vi "AuthSrpInitiationRequest_Parse.vi"(8 "error in (no error)":errorcluster, 11 "Message":T5) -> (0 "error out":errorcluster, 1 "Body":T1, 2 "Header":T3, 3 "AuthSrpInitiationRequest":T2)   [LabVIEW 2017]
uses:
  <vilib>/addons/InsightCM/MessageBus/Base/controls/Message.ctl
  <vilib>/addons/InsightCM/MessageBus/Base/controls/MessageHeader.ctl
  <vilib>/addons/InsightCM/MessageBus/Base/controls/KeyValuePair.ctl
  <vilib>/addons/InsightCM/MessageBus/MessageLibrary/Authentication/controls/AuthSrpInitiationRequest.ctl
  <vilib>/addons/InsightCM/MessageBus/MessageLibrary/Authentication/controls/AuthSrpInitiationRequestBody.ctl
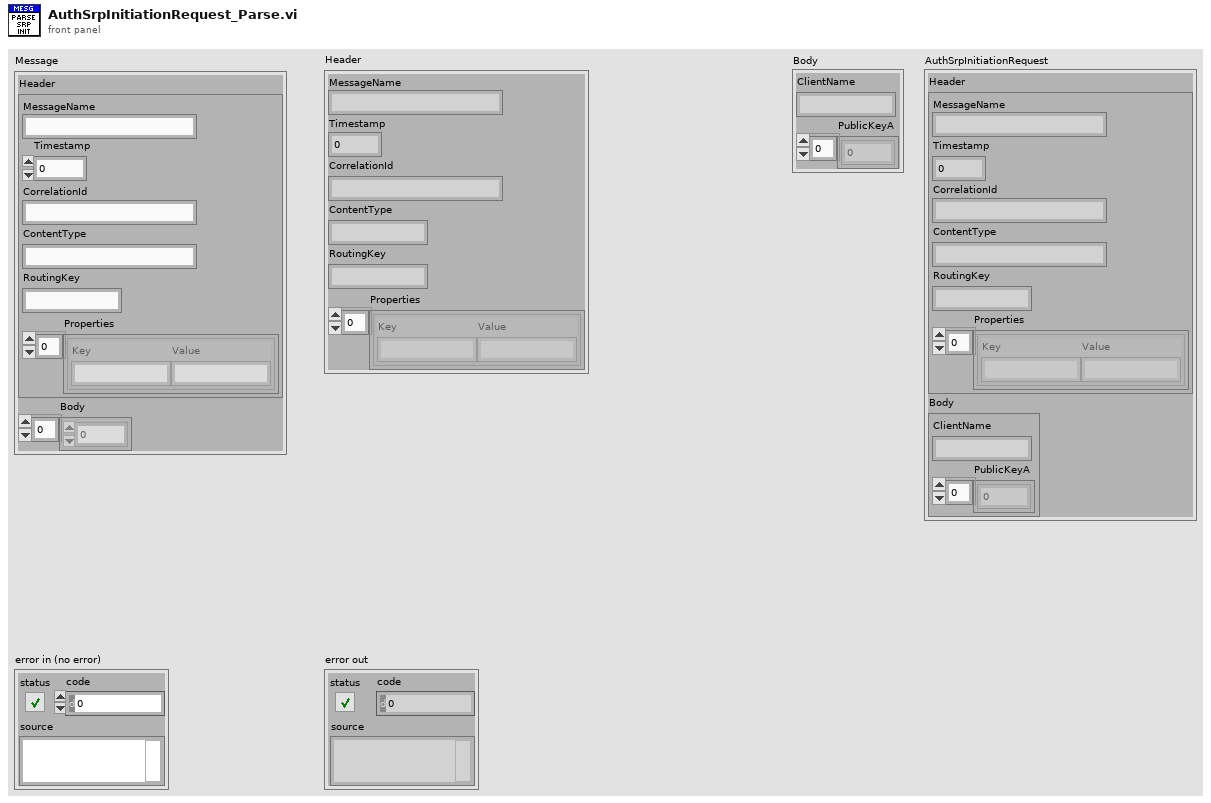
[diagram p1: front panel]
types:
  T1 = typedef "AuthSrpInitiationRequestBody.ctl" = cluster{"ClientName":string, "PublicKeyA":u8[]}
  T2 = typedef "AuthSrpInitiationRequest.ctl" = cluster{"Header":T3, "Body":T1}
  T3 = typedef "MessageHeader.ctl" = cluster{"MessageName":string, "Timestamp":i64, "CorrelationId":string, "ContentType":string, "RoutingKey":string, "Properties":T4[]}
  T4 = typedef "KeyValuePair.ctl" = cluster{"Key":string, "Value":string}
  T5 = typedef "Message.ctl" = cluster{"Header":T3, "Body":u8[]}
  T6 = cluster{"ClientName":string, "PublicKeyA":string}
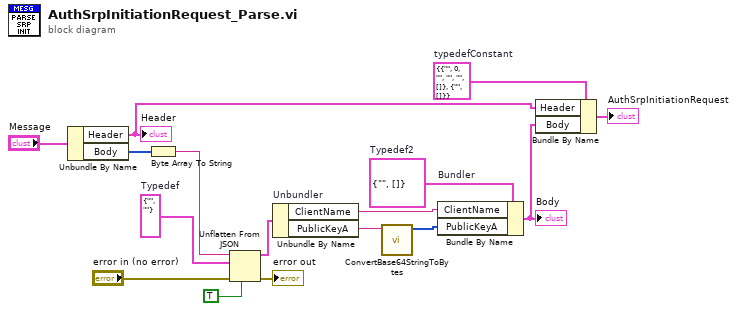
[diagram p0: block diagram]
diagram:
  w4 = T1 {"ClientName"="", "PublicKeyA"=[]}  # Typedef2
  w8 = T2 {"Header"={"MessageName"="", "Timestamp"=0, "CorrelationId"="", "ContentType"="", "RoutingKey"="", "Properties"=[]}, "Body"={"ClientName"="", "PublicKeyA"=[]}}  # typedefConstant
  w12 = T6 {"ClientName"="", "PublicKeyA"=""}  # Typedef
  n1 = Unbundle By Name("Message") -> ("Header"=w14:T3, "Body"=w6:u8[])
  "Header" <- w14
  n2 = Byte Array To String(unsigned byte array=w6) -> (string=w11:string)
  n3 = Unflatten From JSON(JSON string=w11, type and defaults=w12, default null elements? (F)=TRUE, error in (no error)="error in (no error)") -> (value=w10:T6, error out=→"error out":errorcluster)  [unwired: 3 in]
  n4 = Unbundle By Name "Unbundler"(w10) -> ("ClientName"=w3:string, "PublicKeyA"=w2:string)
  n5 = call <vilib>:"ConvertBase64StringToBytes.vi"("Base64 string"=w2) -> ("U8 array"=w1:u8[])  [unwired: 9 in, 1 out]
  n6 = Bundle By Name "Bundler"(cluster=w4, "ClientName"=w3, "PublicKeyA"=w1) -> (w5:T1)
  "Body" <- w5
  n7 = Bundle By Name(cluster=w8, "Header"=w14, "Body"=w5) -> (→"AuthSrpInitiationRequest":T2)
